vi "init.vi"(8 "error in (no error)":errorcluster, 11 "Soda Actor in":refnum<class "Soda Actor.lvclass">) -> (0 "error out":errorcluster, 3 "Soda Actor out":refnum<class "Soda Actor.lvclass">)   [LabVIEW 2019, in "Soda Actor.lvlib" / "Soda Actor.lvclass"]
uses:
  Soda Actor.lvclass
  Soda Actor.lvclass/Soda Actor.ctl
  <vilib>/Utility/config.llb/Write Key (String).vi
  <vilib>/Utility/config.llb/NI_LVConfig.lvlib
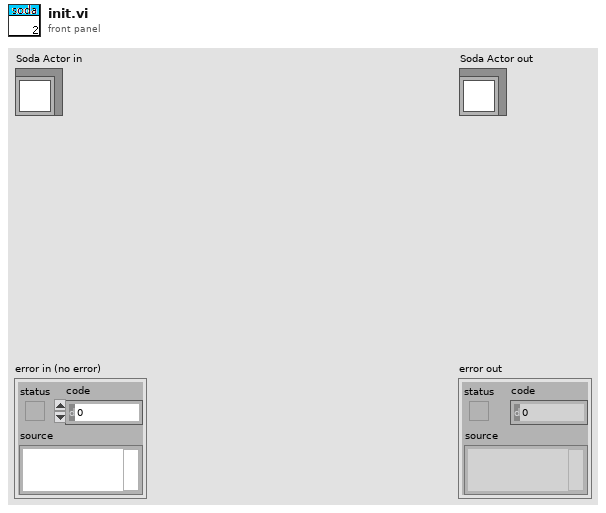
[diagram p1: front panel]
types:
  T1 = typedef "NI_LVConfig.lvlib/Config Data RefNum.ctl" = refnum<k1>
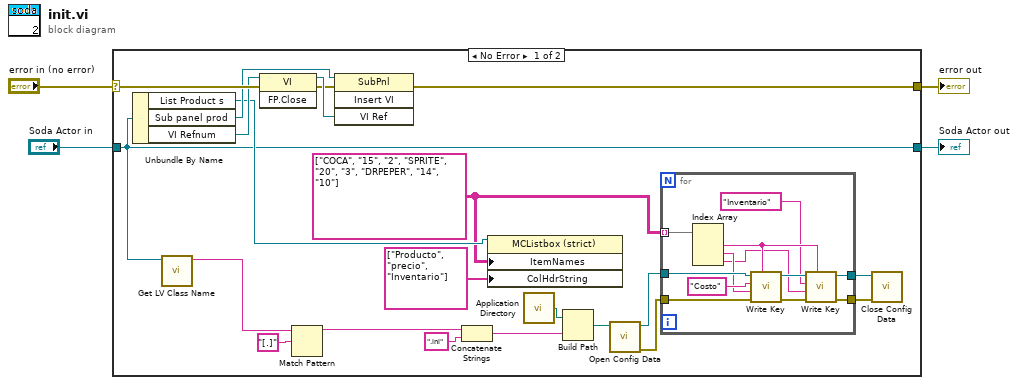
[diagram p0: block diagram]
diagram:
  n1 = case shown="No Error" "error in (no error)" {
    selector: "error in (no error)" -> [w24 w39]
    tunnel: [w20 w39] -> w3
    tunnel: [w17 w38] -> w1
    tunnel: "Soda Actor in" -> [w17 w38]
    frame No Error {
      w12 = string[][] [["COCA", "15", "2"], ["SPRITE", "20", "3"], ["DRPEPER", "14", "10"]] ("Item Names")
      n2 = Unbundle By Name(w17) -> ("List Product s"=w19:refnum<vi>, "Sub panel prod"=w22:refnum<vi>, "VI Refnum"=w23:refnum<vi>)
      n3 = call <vilib>:"Get LV Class Name.vi"("object"=w17) -> ("class name"=w7:string)  [unwired: 9 in, 1 out]
      n4 = invoke class="VI" method="FP.Close"(reference=w23, error in=w24) -> (reference out=w25:refnum<vi>, error out=w21:errorcluster)  [unwired: 1 in, 1 out]
      n5 = Match Pattern(string=w7, regular expression="[.]") -> (before substring=w5:string)  [unwired: 1 in, 3 out]
      n6 = invoke class="SubPnl" method="Insert VI"(reference=w22, error in=w21, "VI Ref"=w25) -> (error out=w20:errorcluster)  [unwired: 1 in, 3 out]
      n7 = Concatenate Strings(w5, ".ini" ("string")) -> (w15:string)
      n8 = property class="MCListbox (strict)"(reference=w19, "ItemNames"=w12, "ColHdrString"=string[] ["Producto", "precio", "Inventario"] ("Column Header Strings[]")) -> ()  [unwired: 1 in, 2 out]
      n9 = call <vilib>:"Application Directory.vi"() -> ("Application Directory"=w16:path)
      n10 = Build Path(base path=w16, name or relative path=w15) -> (appended path=w13:path)
      n11 = call <vilib>:"Open Config Data.vi"("configuration file path"=w13) -> ("error out"=w11:errorcluster, "refnum"=w10:T1)  [unwired: 8 in, 1 out]
      n12 = for {
        tunnel: w12 -> [w31] mode=indexing
        tunnel: w11 -> [w36]
        tunnel: w10 -> [w37]
        tunnel: [w33] -> w8
        tunnel: [w32] -> w9
        n13 = Index Array(array=w31) -> (element #1=w30:string, element #2=w27:string, element #3=w26:string)  [unwired: 3 in]
        n14 = call-poly <vilib>:"Write Key.vi"("section"=w30, "error in (no error)"=w36, "value"=w27, "key"="Costo" ("section"), "refnum"=w37) -> ("error out"=w35:errorcluster, "refnum out"=w34:T1)  [unwired: 4 in, 1 out]
        n15 = call-poly <vilib>:"Write Key.vi"("section"=w30, "error in (no error)"=w35, "value"=w26, "key"="Inventario" ("section"), "refnum"=w34) -> ("error out"=w33:errorcluster, "refnum out"=w32:T1)  [unwired: 4 in, 1 out]
      }
      n16 = call <vilib>:"Close Config Data.vi"("error in (no error)"=w8, "refnum"=w9) -> ()  [unwired: 8 in, 2 out]
    }
    frame Error {
    }
  }
  "error out" <- w3
  "Soda Actor out" <- w1
